vi "main.vi"() -> ()   [LabVIEW 2019, in "RT_Game.lvlib" / "Engine.lvclass"]
uses:
  Engine.lvclass
  Globals.vi
  <vilib>/Utility/error.llb/Error Cluster From Error Code.vi
  <vilib>/ErrorRing/Error Ring.xnode
  <vilib>/NI_Real-Time Target Support.lvlib
panel:
  in  "AttractMode":bool
  in  "SimulateError":bool
  out "delta t":dbl(graph)=11.0
  out "cpu":cluster{"Total (%)":dbl, "Total (%)":dbl}(graph)={"Total (%)"=36.40655155071103, "Total (%)"=28.773757553198372}
  in  "Stop":bool
  out "Error Out":errorcluster
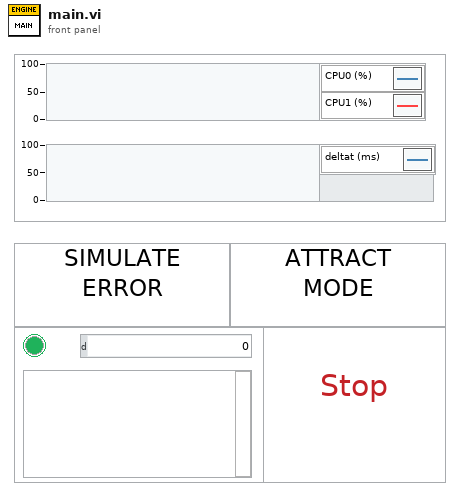
[diagram p1: front panel]
types:
  T1 = typedef "NI_Real-Time Target Support.lvlib/RT CPU Load.ctl" = cluster{"Total (%)":dbl, "Time Critical (%)":dbl, "Timed Structures (%)":dbl, "High (%)":dbl, "Above Normal (%)":dbl, "Normal (%)":dbl, "Background (%)":dbl, "Idle (%)":dbl, "ISR (%)":dbl}
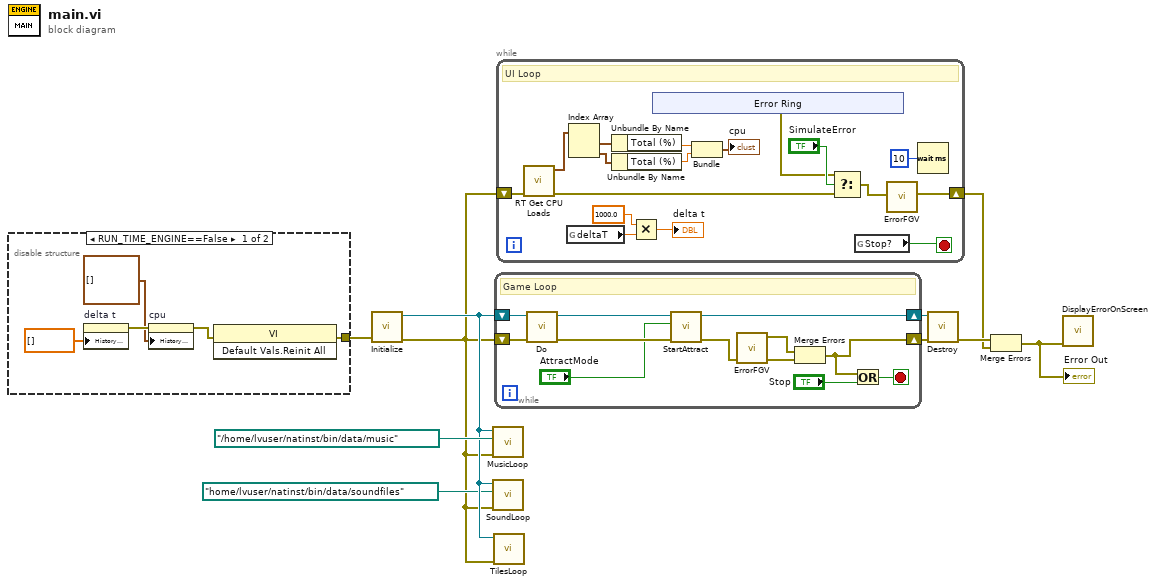
[diagram p0: block diagram]
diagram:
  n1 = disable-structure shown="RUN_TIME_ENGINE==False" {
    disable-tunnel: [w15 _] -> w5
    frame condition #0 (active) {
      n2 = property on="delta t" class="WFChart (strict)"("History Data"=dbl[] []) -> (error out=w13:errorcluster)  [unwired: 2 in, 1 out]
      n3 = property on="cpu" class="WFChart (strict)"(error in=w13, "History Data"=cluster{"Total (%)":dbl, "Total (%)":dbl}[] []) -> (error out=w14:errorcluster)  [unwired: 1 in, 1 out]
      n4 = invoke class="VI" method="Default Vals.Reinit All"(error in=w14) -> (error out=w15:errorcluster)  [unwired: 2 in, 2 out]
    }
    frame condition #1 {
    }
  }
  n5 = call "Initialize.vi"("error in (no error)"=w5) -> ("error out"=w3:errorcluster, "Engine out"=w7:refnum<class "Engine.lvclass">)  [unwired: 9 in]
  n6 = call "MusicLoop.vi"("error in (no error)"=w3, "Tracks"=path "//home/lvuser/natinst/bin/data/music", "Engine in"=w7) -> ()  [unwired: 8 in, 1 out]
  n7 = call "SoundLoop.vi"("error in (no error)"=w3, "SoundsFolder"=path "/home/lvuser/natinst/bin/data/soundfiles", "Engine in"=w7) -> ()  [unwired: 8 in, 1 out]
  n8 = call "TilesLoop.vi"("error in (no error)"=w3, "Engine in"=w7) -> ()  [unwired: 9 in, 1 out]
  n9 = while {
    shift-right: [w17] -> w10
    shift-left: w7 -> [w26]
    shift-right: [w22] -> w9
    shift-left: w3 -> [w25]
    stop <- w24 stop-if-true
    # "Game Loop"
    n10 = call "Do.vi"("error in (no error)"=w25, "Engine in"=w26) -> ("error out"=w23:errorcluster, "Engine out"=w18:refnum<class "Engine.lvclass">)  [unwired: 8 in]
    n11 = call "StartAttract.vi"("error in (no error)"=w23, "Start?"="AttractMode", "Engine in"=w18) -> ("error out"=w19:errorcluster, "Engine out"=w17:refnum<class "Engine.lvclass">)  [unwired: 7 in]
    n12 = call "ErrorFGV.vi"() -> ("SlaveLoopError"=w21:errorcluster)  [unwired: 10 in, 1 out]
    n13 = Merge Errors(w21, w19) -> (w22:errorcluster)
    n14 = Or(x=w22, y="Stop") -> (x .or. y?=w24:bool)
  }
  n15 = while {
    shift-right: [w36] -> w1
    shift-left: w3 -> [w37]
    stop <- w27 stop-if-true
    # "UI Loop"
    n16 = call <vilib>:"RT Get CPU Loads.vi"("error in (no error)"=w37) -> ("error out"=w30:errorcluster, "CPU loads"=w40:T1[])  [unwired: 9 in]
    n17 = global read "Globals.vi" "deltaT"() -> (w43:dbl)
    n18 = Index Array(array=w40) -> (element #1=w41:T1, element #2=w42:T1)  [unwired: 2 in]
    n19 = Unbundle By Name(w41) -> ("Total (%)"=w35:dbl)
    n20 = Unbundle By Name(w42) -> ("Total (%)"=w34:dbl)
    n21 = Multiply(x=1000.0, y=w43) -> (x*y=→"delta t":dbl)
    n22 = xnode "Error Ring"() -> ("error out"=w28:errorcluster)
    n23 = Bundle("Total (%)"=w35, "Total (%)"=w34) -> (→"cpu":cluster{"Total (%)":dbl, "Total (%)":dbl})  [unwired: 1 in]
    n24 = Select(t=w28, s="SimulateError", f=w30) -> (s? t:f=w31:errorcluster)
    n25 = global read "Globals.vi" "Stop?"() -> (w27:bool)
    n26 = call "ErrorFGV.vi"("error in (no error)"=w31) -> ("error out"=w36:errorcluster)  [unwired: 9 in, 1 out]
    n27 = Wait (ms)(milliseconds to wait=u32 10) -> ()  [unwired: 1 out]
  }
  n28 = call "Destroy.vi"("error in (no error)"=w9, "Engine in"=w10) -> ("error out"=w4:errorcluster)  [unwired: 9 in]
  n29 = Merge Errors(w4, w1) -> (w2:errorcluster)
  "Error Out" <- w2
  n30 = call "DisplayErrorOnScreen.vi"("error in (no error)"=w2) -> ()  [unwired: 11 in]
